vi "3.2.1-VectorNav.vi"(0 "error in":errorcluster, 1 "FPGA Ref In":T1) -> (2 "Data":dbl[](array[numeric]), 3 "error out":errorcluster, 4 "FPGA Ref Out":T1)   [LabVIEW 2010]
doc: "This VI demonstrates simple on-demand sampling of a serial port module. It communicates string commands and reads replies via DMA FIFOs, and uses boolean flags to signal to the FPGA when to read and write to those FIFOs. This is necessary because the FPGA runs much faster than the cRIO, so if left to its own devices it would empty the command FIFO and fill up the reply FIFO too quickly.\n\nEvery time the VI is run, it writes a command to a DMA FIFO that it shares with the FPGA, waits for the FPGA to write the command to the VectorNav and read the VectorNav's reply, then reads the FPGA's reply from a second DMA FIFO. It then parses the reply and updates global variables accordingly."
uses:
  3.2.1-VectorNav Registers.ctl
  2-Low Neurons/2-FPGA VI Typedef.ctl
  3.0-Global.vi
panel:
  out "Register":T2
  out "Header":string
  out "Reading":bool=TRUE
  out "Waiting":bool=TRUE
  out "Writing":bool=TRUE
  out "Reply":string
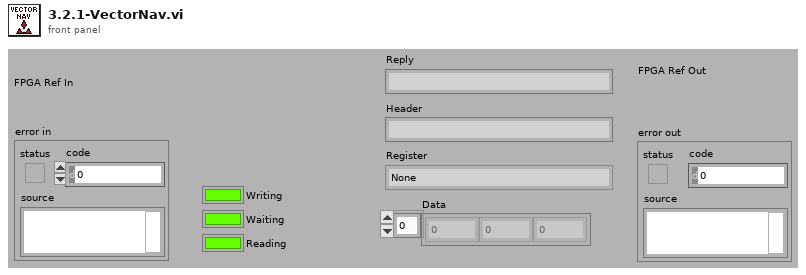
[diagram p1: front panel]
types:
  T1 = typedef "2-FPGA VI Typedef.ctl" = refnum<k20>
  T2 = typedef "3.2.1-VectorNav Registers.ctl" = enum16{"None", "Model Number", "Hardware Revision", "Serial Number", "Firmware Version", "Serial Baud Rate", "Async Data Output Type", "Async Data Output Freq", "Attitude (Yaw, Pitch, Roll)", "Attitude (Quaternion)"}
  T3 = typedef "3.2.1-VectorNav Command Type.ctl" = cluster{"Command type":enum16{"Attitude (Yaw, Pitch, Roll)", "Write Current Settings", "Disable Async Output", "Tare", "Manual"}, "Manual command":string}
  T4 = enum16{"Attitude (Yaw, Pitch, Roll)", "Write Current Settings", "Disable Async Output", "Tare", "Manual"}
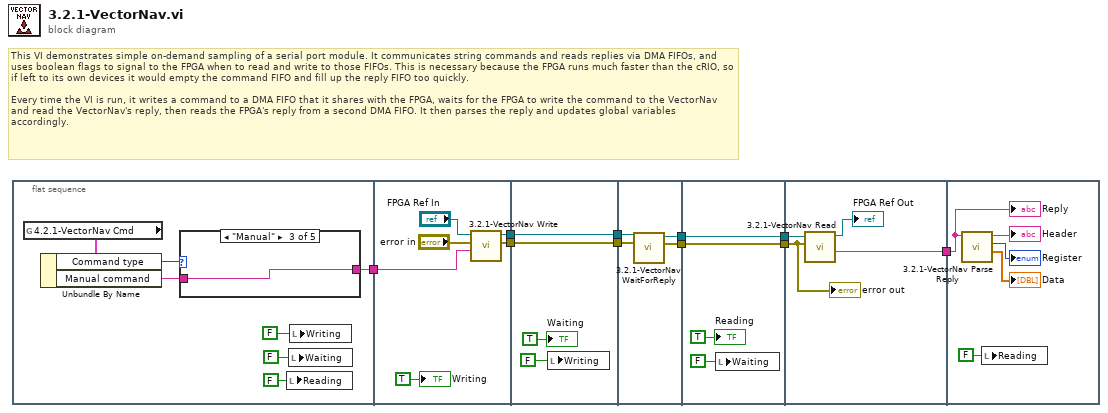
[diagram p0: block diagram]
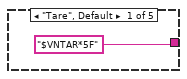
[diagram p2: hidden frame]
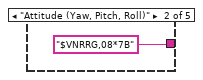
[diagram p3: hidden frame]
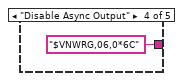
[diagram p4: hidden frame]
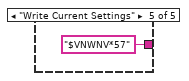
[diagram p5: hidden frame]
diagram:
  # "This VI demonstrates simple on-demand sampling of a serial port module. It communicates string commands and reads replies via DMA FIFOs, and uses boolean flags to signal to the FPGA when to read and write to those FIFOs. This is necessary because the FPGA runs much faster than the cRIO, so if left to its own devices it would empty the command FIFO and fill up the reply FIFO too quickly.\n\nEvery time the VI is run, it writes a command to a DMA FIFO that it shares with the FPGA, waits for the FPGA to write the command to the VectorNav and read the VectorNav's reply, then reads the FPGA's reply from a second DMA FIFO. It then parses the reply and updates global variables accordingly."
  n1 = flat-sequence {
    tunnel: [w14] -> w1
    tunnel: [w28] -> w10
    tunnel: [w27] -> w8
    tunnel: w1 -> [w25]
    tunnel: w10 -> [w32]
    tunnel: [w32] -> w9
    tunnel: w8 -> [w31]
    tunnel: [w31] -> w7
    tunnel: w9 -> [w35]
    tunnel: w7 -> [w36]
    tunnel: [w34] -> w6
    tunnel: [w33] -> w4
    tunnel: w6 -> [w40]
    tunnel: [w40] -> w5
    tunnel: w4 -> [w39]
    tunnel: [w39] -> w3
    tunnel: w5 -> [w41]
    tunnel: w3 -> [w44]
    tunnel: [w43] -> w2
    tunnel: w2 -> [w46]
    frame #0 {
      n2 = global read "3.0-Global.vi" "4.2.1-VectorNav Cmd"() -> (w13:T3)
      n3 = Unbundle By Name(w13) -> ("Command type"=w12:T4, "Manual command"=w11:string)
      n4 = case shown="\"Manual\"" w12 {
        tunnel: ["$VNTAR*5F" "$VNRRG,08*7B" w20 "$VNWRG,06,0*6C" ("Manual command") "$VNWNV*57" ("Manual command")] -> w14
        tunnel: w11 -> [_ _ w20 _ _]
        frame "Tare", Default {
        }
        frame "Attitude (Yaw, Pitch, Roll)" {
        }
        frame "Manual" {
        }
        frame "Disable Async Output" {
        }
        frame "Write Current Settings" {
        }
      }
      n5 = local write "Reading"(FALSE ("Writing")) -> ()
      n6 = local write "Waiting"(FALSE ("Writing")) -> ()
      n7 = local write "Writing"(FALSE ("Writing")) -> ()
    }
    frame #1 {
      n8 = call "3.2.1-VectorNav Write.vi"("Command"=w25, "error in"="error in", "FPGA Ref In"="FPGA Ref In") -> ("error out"=w27:errorcluster, "FPGA VI Reference Out"=w28:T1)  [unwired: 7 in]
      "Writing" <- TRUE
    }
    frame #2 {
      n9 = local write "Writing"(FALSE ("Writing")) -> ()
      "Waiting" <- TRUE
    }
    frame #3 {
      n10 = call "3.2.1-VectorNav WaitForReply.vi"("error in"=w36, "FPGA Ref In"=w35) -> ("error out"=w34:errorcluster, "FPGA Ref Out"=w33:T1)  [unwired: 8 in]
    }
    frame #4 {
      n11 = local write "Waiting"(FALSE ("Writing")) -> ()
      "Reading" <- TRUE
    }
    frame #5 {
      n12 = call "3.2.1-VectorNav Read.vi"("error in"=w41, "FPGA Ref In"=w44) -> ("Final Reply"=w43:string, "FPGA VI Reference Out"=→"FPGA Ref Out":T1)  [unwired: 7 in, 1 out]
      "error out" <- w41
    }
    frame #6 {
      n13 = call "3.2.1-VectorNav Parse Reply.vi"("Input String"=w46) -> ("Data"=→"Data":dbl[], "Register"=→"Register":T2, "Header"=→"Header":string)  [unwired: 8 in]
      n14 = local write "Reading"(FALSE ("Writing")) -> ()
      "Reply" <- w46
    }
  }
